vi "Image Coordinet.vi"(9 "Out":T1(array[cluster]), 10 "index of element":i32, 11 "Picture in":refnum<vi>) -> ()   [LabVIEW 2015]
uses:
  <vilib>/Utility/miscctls.llb/LVPointTypeDef.ctl
  <vilib>/Utility/miscctls.llb/LVBoundsTypeDef.ctl
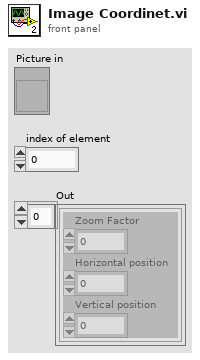
[diagram p1: front panel]
types:
  T1 = cluster{"Zoom Factor":sgl, "Horizontal position":sgl, "Vertical position":sgl}[]
  T2 = typedef "LVBoundsTypeDef.ctl" = cluster{"Width":u32, "Height":u32}
  T3 = typedef "LVPointTypeDef.ctl" = cluster{"Horizontal":i16, "Vertical":i16}
  T4 = cluster{"Zoom Factor":sgl, "Horizontal position":sgl, "Vertical position":sgl}
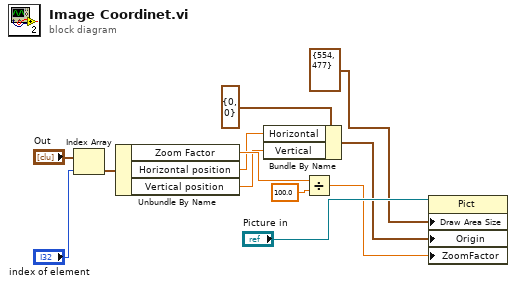
[diagram p0: block diagram]
diagram:
  n1 = Index Array(array="Out", index="index of element") -> (element=w4:T4)
  n2 = Unbundle By Name(w4) -> ("Zoom Factor"=w8:sgl, "Horizontal position"=w2:sgl, "Vertical position"=w1:sgl)
  n3 = Bundle By Name(cluster=T3 {"Horizontal"=0, "Vertical"=0} ("Origin"), "Horizontal"=w2, "Vertical"=w1) -> (w10:T3)
  n4 = Divide(x=w8, y=sgl 100.0 ("x")) -> (x/y=w11:sgl)
  n5 = property class="Pict"(reference="Picture in", "Draw Area Size"=T2 {"Width"=554, "Height"=477}, "Origin"=w10, "ZoomFactor"=w11) -> ()  [unwired: 1 in, 2 out]
